vi "Find Prefix.vi"(9 "--X":T1, 10 "VI Ref":refnum<vi>) -> (2 "Prefix":string)   [LabVIEW 2025, in "jettl.lvlib" / "Actor.lvlib"]
uses:
  Actor.lvlib
  --X.ctl
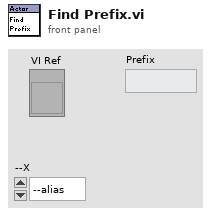
[diagram p1: front panel]
types:
  T1 = typedef "jettl.lvlib/Actor.lvlib/--X.ctl" = enum16{"--alias", "--create", "--error"}
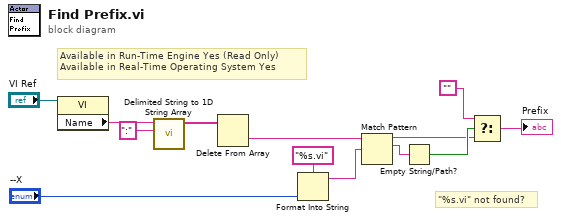
[diagram p0: block diagram]
diagram:
  # "Available in Run-Time Engine Yes (Read Only) \nAvailable in Real-Time Operating System Yes"
  # "\"%s.vi\" not found?"
  n1 = property class="VI"(reference="VI Ref") -> ("Name"=w1:string)  [unwired: 1 in, 2 out]
  n2 = call <vilib>:"Delimited String to 1D String Array.vi"("delimiter"=":", "delimited string"=w1) -> ("string array"=w11:string[])  [unwired: 9 in]
  n3 = Delete From Array "Delete From Array"(array=w11) -> (deleted portion=w10:string)  [unwired: 2 in, 1 out]
  n4 = Format Into String(format string="%s.vi" ("regular expression"), "--X") -> (resulting string=w4:string)  [unwired: 2 in, 1 out]
  n5 = Match Pattern(string=w10, regular expression=w4) -> (before substring=w7:string, match substring=w13:string)  [unwired: 1 in, 2 out]
  n6 = Empty String/Path?(string/path=w13) -> (empty?=w8:bool)
  n7 = Select(t="", s=w8, f=w7) -> (s? t:f=→"Prefix":string)
